vi "Grab.vi"(8 "error in (no error)":errorcluster, 10 "Image":T1, 11 "Sim Camera Driver in":refnum<class "Sim Camera Driver.lvclass">) -> (0 "error out":errorcluster, 2 "Image out":T1, 3 "Sim Camera Driver out":refnum<class "Sim Camera Driver.lvclass">)   [LabVIEW 2022 SP3, in "Sim Camera Driver.lvclass"]
uses:
  Sim Camera Driver.lvclass
  <vilib>/vision/Image Controls.llb/IMAQ Image.ctl
  Sim Camera Driver.lvclass/Sim Camera Driver.ctl
  <vilib>/Utility/file.llb/Read Delimited Spreadsheet (I64).vi
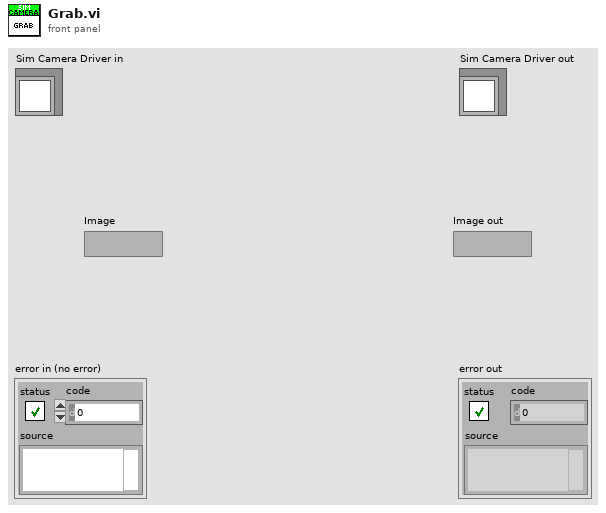
[diagram p1: front panel]
types:
  T1 = typedef "IMAQ Image.ctl" = refnum<image>
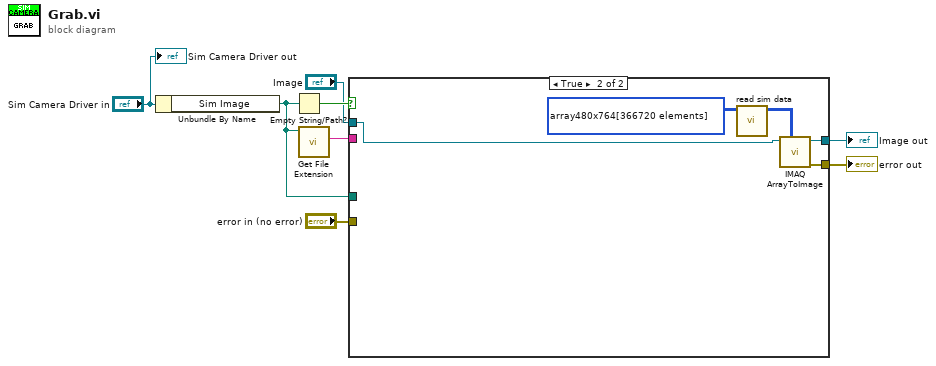
[diagram p0: block diagram]
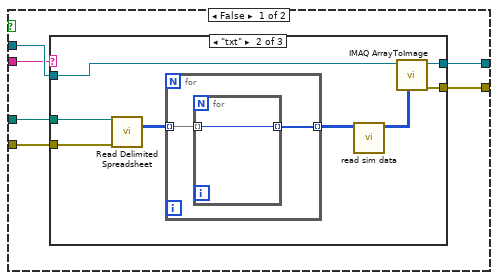
[diagram p2: hidden frame]
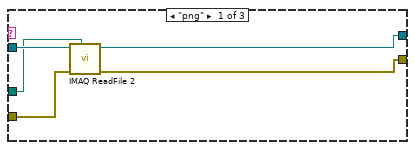
[diagram p3: hidden frame]
diagram:
  n1 = Unbundle By Name("Sim Camera Driver in") -> ("Sim Image"=w4:path)
  n2 = Empty String/Path?(string/path=w4) -> (empty?=w2:bool)
  n3 = call <vilib>:"Get File Extension.vi"("file"=w4) -> ("lowercase file extension"=w6:string)  [unwired: 6 in, 4 out]
  n4 = case shown="True" w2 {
    tunnel: "Image" -> [w14 w35]
    tunnel: [w13 w37] -> w7
    tunnel: w6 -> [w12 _]
    tunnel: [w11 w36] -> w5
    tunnel: w4 -> [w10 _]
    tunnel: "error in (no error)" -> [w9 _]
    frame False {
      n5 = case shown="\"txt\"" w12 {
        tunnel: w9 -> [w16 w27 w31]
        tunnel: w10 -> [w18 w26 _]
        tunnel: w14 -> [w19 w24 w32]
        tunnel: [w15 w23 w31] -> w11
        tunnel: [w17 w22 w32] -> w13
        frame "png" {
          n6 = call "IMAQ ReadFile 2"("File Path"=w18, "error in (no error)"=w16, "Image"=w19) -> ("error out"=w15:errorcluster, "Image Out"=w17:T1)  [unwired: 4 in, 3 out]
        }
        frame "txt" {
          n7 = call-poly <vilib>:"Read Delimited Spreadsheet.vi"("file path (dialog if empty)"=w26, "error in (no error)"=w27) -> ("all rows"=w21:i64[][])  [unwired: 8 in, 5 out]
          n8 = for {
            tunnel: w21 -> [w29] mode=indexing
            tunnel: [w28] -> w20 mode=indexing
            n9 = for {
              tunnel: w29 -> [w30] mode=indexing
              tunnel: [w30] -> w28 mode=indexing
            }
          }
          n10 = call "read sim data.vi"("Array IN"=w20) -> ("Array Out"=w25:u16[][])  [unwired: 10 in]
          n11 = call "IMAQ ArrayToImage"("Image Pixels (Float)"=w25, "Image"=w24) -> ("error out"=w23:errorcluster, "Image Out"=w22:T1)  [unwired: 8 in]
        }
        frame Default {
        }
      }
    }
    frame True {
      n12 = call "read sim data.vi"("Array IN"=u16[][] array480x764[366720 elements] ("Array")) -> ("Array Out"=w33:u16[][])  [unwired: 10 in]
      n13 = call "IMAQ ArrayToImage"("Image Pixels (U16)"=w33, "Image"=w35) -> ("error out"=w36:errorcluster, "Image Out"=w37:T1)  [unwired: 8 in]
    }
  }
  "error out" <- w5
  "Image out" <- w7
  "Sim Camera Driver out" <- "Sim Camera Driver in"
